vi "DisableChangeDTCsCount.vi"(8 "error in (no error)":errorcluster, 11 "connection info":T1) -> (0 "error out":errorcluster, 3 "connection info":T1)   [LabVIEW 2015, in "Diagnostics Host Automation API.lvlib"]
uses:
  Diagnostics Host Automation API.lvlib
  <vilib>/NI/STM/TCP/TCP Connection Info.ctl
  <vilib>/NI/STM/SubVIs/MetaDataElement.ctl
  <vilib>/NI/NIVS Addon Network Comm/Shared/NI VeriStand Addon Network Comm Shared.lvlib
  <vilib>/NI/STM/NI STM.lvlib
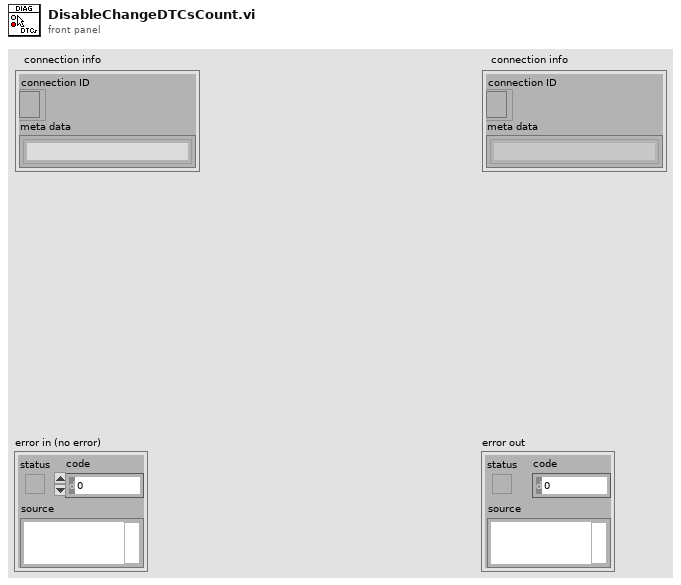
[diagram p1: front panel]
types:
  T1 = typedef "NI STM.lvlib/TCP Connection Info.ctl" = cluster{"connection ID":refnum<k5>, "meta data":T2[]}
  T2 = typedef "NI STM.lvlib/MetaDataElement.ctl" = string
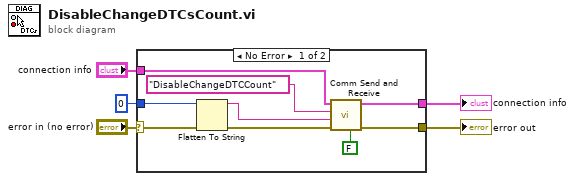
[diagram p0: block diagram]
diagram:
  n1 = case shown="No Error" "error in (no error)" {
    selector: "error in (no error)" -> [w10 w16]
    tunnel: "connection info" -> [w14 w15]
    tunnel: [w13 w15] -> w4
    tunnel: [w12 w16] -> w3
    tunnel: u8 0 ("status mask") -> [w7 _]
    frame No Error {
      n2 = Flatten To String(anything=w7, error in (no error)=w10) -> (data string=w8:string, error out=w9:errorcluster)  [unwired: 2 in, 1 out]
      n3 = call <vilib>:"Comm Send and Receive.vi"("Resp Required?"=FALSE, "error in (no error)"=w9, "Data"=w8, "Name"="DisableChangeDTCCount", "connection info"=w14) -> ("error out"=w12:errorcluster, "connection info"=w13:T1)  [unwired: 3 in, 2 out]
    }
    frame Error {
    }
  }
  "connection info" <- w4
  "error out" <- w3
